vi "gun_speed_control P2ID.vi"(9 "Period (sec)":dbl, 10 "Speed (rps)":dbl, 11 "Gun Const":T1={"gun"={"num_lines"=0.0, "gain_kp1"=0.0, "gain_kp2"=0.0, "gain_ki"=0.0, "gain_kd"=0.0}, "turret"={"center_ana"=0.0, "volts_per_180"=0.0, "man_scale"=0.0, "turret_idg"={"low_fault_ana"=0.0, "high_fault_ana"=0.0, "min_ana"=0.0, "max_ana"=0.0, "movement_thresh"=0.0, "movement_time"=0.0}, "turret_pid"={"kP"=0.0, "kI"=0.0, "kD"=0.0}, "turret_invert"=TRUE, "turret_low_power"=0.0}, "tracking"={"velocity_lead_gain"=0.0, "velocity_rotation_gain"=0.0}, "hood"={"hood_idg"={"low_fault_ana"=0.0, "high_fault_ana"=0.0, "min_ana"=0.0, "max_ana"=0.0, "movement_thresh"=0.0, "movement_time"=0.0}, "hood_pid"={"kP"=0.0, "kI"=0.0, "kD"=0.0}, "hood_scale"={"min_ana"=0.0, "min_units"=0.0, "max_ana"=0.0, "max_units"=0.0}, "hood_invert"=FALSE}}) -> (1 "RPM raw":dbl, 2 "Sensor Speed (rps)":dbl, 3 "Output":dbl)   [LabVIEW 2011]
uses:
  gun_const_t.ctl
  gun_idg_const.ctl
  common/gain_const.ctl
  common/scale_const.ctl
  signals/Signal.ctl
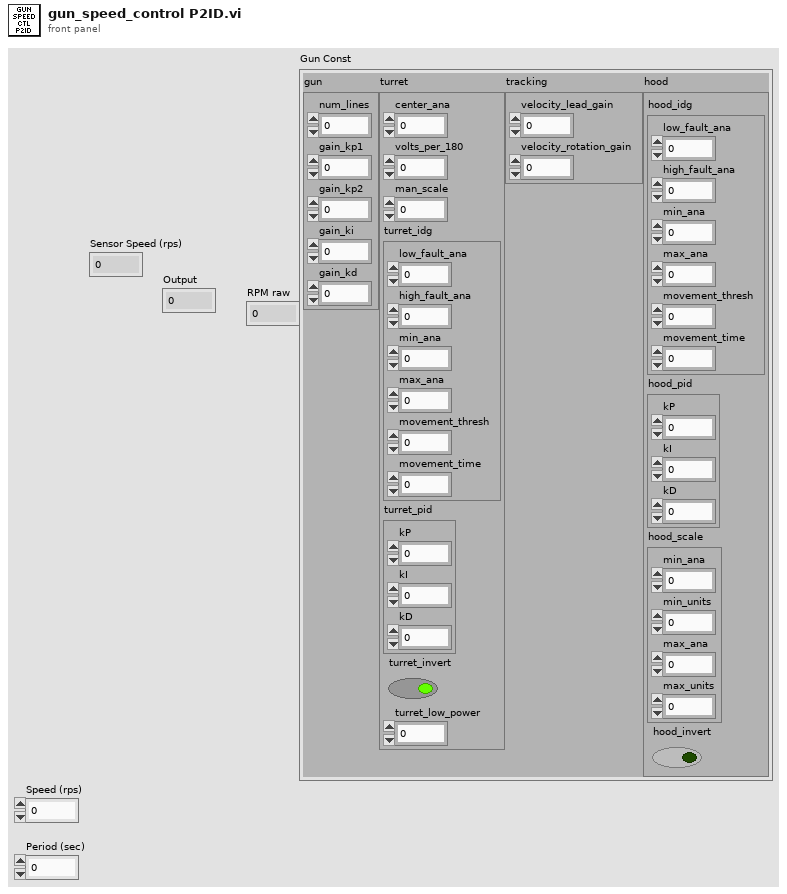
[diagram p1: front panel]
types:
  T1 = typedef "gun_const_t.ctl" = cluster{"gun":cluster{"num_lines":dbl, "gain_kp1":dbl, "gain_kp2":dbl, "gain_ki":dbl, "gain_kd":dbl}, "turret":cluster{"center_ana":dbl, "volts_per_180":dbl, "man_scale":dbl, "turret_idg":T2, "turret_pid":T3, "turret_invert":bool, "turret_low_power":dbl}, "tracking":cluster{"velocity_lead_gain":dbl, "velocity_rotation_gain":dbl}, "hood":cluster{"hood_idg":T2, "hood_pid":T3, "hood_scale":T4, "hood_invert":bool}}
  T2 = typedef "gun_idg_const.ctl" = cluster{"low_fault_ana":dbl, "high_fault_ana":dbl, "min_ana":dbl, "max_ana":dbl, "movement_thresh":dbl, "movement_time":dbl}
  T3 = typedef "gain_const.ctl" = cluster{"kP":dbl, "kI":dbl, "kD":dbl}
  T4 = typedef "scale_const.ctl" = cluster{"min_ana":dbl, "min_units":dbl, "max_ana":dbl, "max_units":dbl}
  T5 = typedef "Signal.ctl" = enum16{"SIGFIRE", "SIGSTOPSCRIPT", "SIGSTARTGUN", "SIGSTOPGUN", "SIGDISABLED", "SIGENABLED", "SIGUDPTIMEOUT", "SIGNEWVISION_REMOTE", "SIGNEWVISION_LOCAL", "SIGSHOTFIRED", "SIGDOTRACK", "SIGDONTTRACK"}
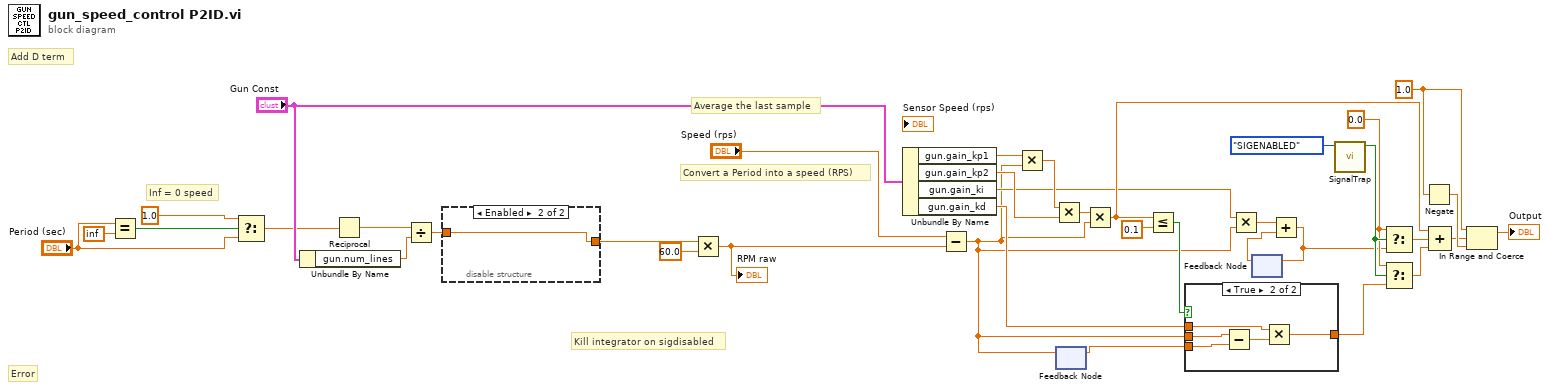
[diagram p0: block diagram]
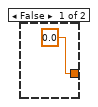
[diagram p2: hidden frame]
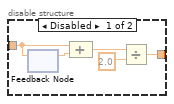
[diagram p3: hidden frame]
diagram:
  w12 = 0.0
  w21 = 1.0
  # "Add D term"
  # "Inf = 0 speed"
  # "Kill integrator on sigdisabled"
  # "Average the last sample"
  # "Error"
  # "Convert a Period into a speed (RPS)"
  n1 = Equal?(x="Period (sec)", y=inf) -> (x = y?=w30:bool)
  n2 = Select(t=1.0, s=w30, f="Period (sec)") -> (s? t:f=w27:dbl)
  n3 = Unbundle By Name("Gun Const") -> ("gun.num_lines"=w37:dbl)
  n4 = Reciprocal(x=w27) -> (1/x=w34:dbl)
  n5 = Divide(x=w34, y=w37) -> (x/y=w36:dbl)
  n6 = disable-structure shown="Enabled" {
    disable-tunnel: w36 -> [w39 w43]
    disable-tunnel: [w38 w43] -> w26
    frame Disabled {
      n7 = feedback #1() -> (w40:dbl)  [unwired: 1 in]
      n8 = feedback-in #1(w39) -> ()
      n9 = Compound Arithmetic op=ADD(w39, w40) -> (w41:dbl)
      n10 = Divide(x=w41, y=2.0) -> (x/y=w38:dbl)
    }
    frame Enabled {
    }
  }
  n11 = Multiply(x=w26, y=60.0) -> (x*y=w2:dbl)
  "RPM raw" <- w2
  n12 = Unbundle By Name("Gun Const") -> ("gun.gain_kp1"=w25:dbl, "gun.gain_kp2"=w10:dbl, "gun.gain_ki"=w5:dbl, "gun.gain_kd"=w17:dbl)
  n13 = Subtract(x="Speed (rps)", y=w2) -> (x-y=w4:dbl)
  n14 = Multiply(x=w25, y=w4) -> (x*y=w9:dbl)
  n15 = Multiply(x=w9, y=w10) -> (x*y=w11:dbl)
  n16 = feedback #2() -> (w8:dbl)  [unwired: 1 in]
  n17 = feedback-in #2(w4) -> ()
  n18 = Multiply(x=w11, y=w4) -> (x*y=w22:dbl)
  n19 = Less Or Equal?(x=w22, y=0.1) -> (x <= y?=w23:bool)
  n20 = case shown="True" w23 {
    tunnel: [0.0 w47] -> w14
    tunnel: w4 -> [_ w45]
    tunnel: w17 -> [_ w48]
    tunnel: w8 -> [_ w46]
    frame False {
    }
    frame True {
      n21 = Subtract(x=w45, y=w46) -> (x-y=w49:dbl)
      n22 = Multiply(x=w48, y=w49) -> (x*y=w47:dbl)
    }
  }
  n23 = Multiply(x=w5, y=w4) -> (x*y=w7:dbl)
  n24 = feedback #3() -> (w6:dbl)  [unwired: 1 in]
  n25 = Add(x=w7, y=w6) -> (x+y=w3:dbl)
  n26 = feedback-in #3(w3) -> ()
  n27 = call "SignalTrap.vi"("Signal"=Signal."SIGENABLED") -> ("Trapped Signal"=w13:bool)  [unwired: 10 in]
  n28 = Select(t=w12, s=w13, f=w3) -> (s? t:f=w16:dbl)
  n29 = Select(t=w12, s=w13, f=w14) -> (s? t:f=w15:dbl)
  n30 = Negate(x=w21) -> (-x=w20:dbl)
  n31 = Compound Arithmetic op=ADD(w22, w16, w15) -> (w19:dbl)
  n32 = In Range and Coerce(upper limit=w21, x=w19, lower limit=w20) -> (coerced(x)=→"Output":dbl)  [unwired: 1 out]
